vi "Get Child Hwnd.vi"(8 "Error in":errorcluster, 11 "LV Doc.lvclass":refnum<class "LV Doc.lvclass">) -> (0 "Error Out":errorcluster, 3 "LV Doc.lvclass":refnum<class "LV Doc.lvclass">)   [LabVIEW 2016, in "LV Doc.lvclass"]
doc: "Obtain Child window Hwnd."
uses:
  LV Doc.lvclass
  LV Doc.lvclass/LV Doc.ctl
  user32.dll
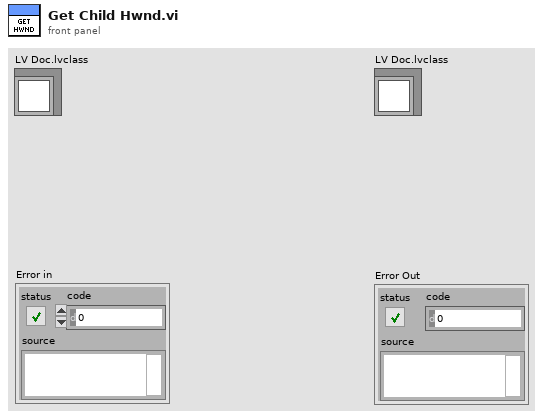
[diagram p1: front panel]
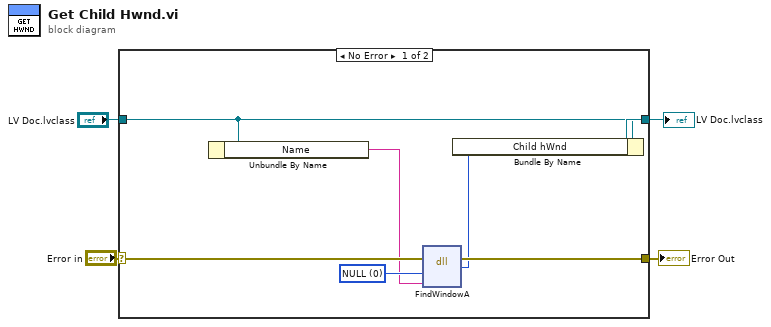
[diagram p0: block diagram]
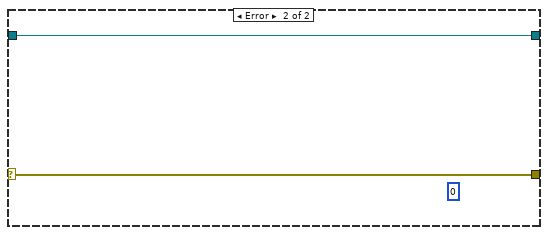
[diagram p2: hidden frame]
diagram:
  n1 = case shown="No Error" "Error in" {
    selector: "Error in" -> [w11 w13]
    tunnel: [w10 w13] -> w3
    tunnel: [w8 w12] -> w1
    tunnel: "LV Doc.lvclass" -> [w7 w12]
    frame No Error {
      w9 = 0 items=["NULL"]
      n2 = Unbundle By Name(w7) -> ("Name"=w6:string)
      n3 = dll-call lib="user32.dll" fn="FindWindowA"(error in=w11, "lpzsClassName"=w9, "lpzsWindowName"=w6) -> (error out=w10:errorcluster, "hwnd"=w5:u32)  [unwired: 4 in, 1 out]
      n4 = Bundle By Name(cluster=w7, "Child hWnd"=w5) -> (w8:refnum<class "LV Doc.lvclass">)
    }
    frame Error {
      (unwired) u32 0 ("hwnd")
    }
  }
  "Error Out" <- w3
  "LV Doc.lvclass" <- w1
